vi "Condition Based on Measurement Result.vi"() -> ()   [LabVIEW 2019]
uses:
  <vilib>/DAQmx/read.llb/DAQmx Read (Analog Wfm 1Chan NSamp).vi
  <vilib>/DAQmx/create/channels.llb/DAQmx Create Channel (AI-Temperature-Thermocouple).vi
  <vilib>/DAQmx/configure/timing.llb/DAQmx Timing (Sample Clock).vi
  <vilib>/DAQmx/miscellaneous.llb/DAQmx Fill In Error Info.vi
  <resource>/objmgr/daqmx.rc
panel:
  in  "Stop":bool
  out "Actual Sample Rate (Hz)":dbl
  in  "DAQmx Physical Channel":tag="PCI-6221/ai1"
  out "Last exceeded temperature":waveform(dbl)(graph)={"t0"=timestamp(3640236029.6826963 s since 1904-01-01), "dt"=0.00039059999999999995, "Y"=array[256 elements], "attributes"=variant("NI_ChannelName"=variant(string "PCI-6221/ai0"), "NI_UnitDescription"=variant(string "Deg C"))}
  out "Current temperature":waveform(dbl)(graph)={"t0"=timestamp(3640236029.6826963 s since 1904-01-01), "dt"=0.00039059999999999995, "Y"=array[256 elements], "attributes"=variant("NI_ChannelName"=variant(string "PCI-6221/ai0"), "NI_UnitDescription"=variant(string "Deg C"))}
  in  "Temperature threshold (C)":dbl=30.0
  in  "Number of Samples":i32=256
  in  "Desired Sample Rate (Hz)":dbl=2560.0
  # "Channel Settings"
  # "______________________________________________"
  # "Timing Settings"
  # "______________________________________________"
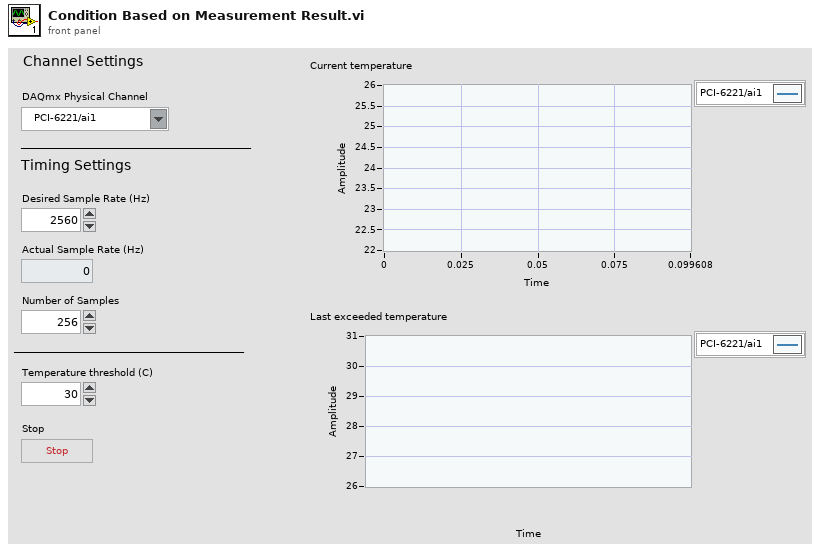
[diagram p1: front panel]
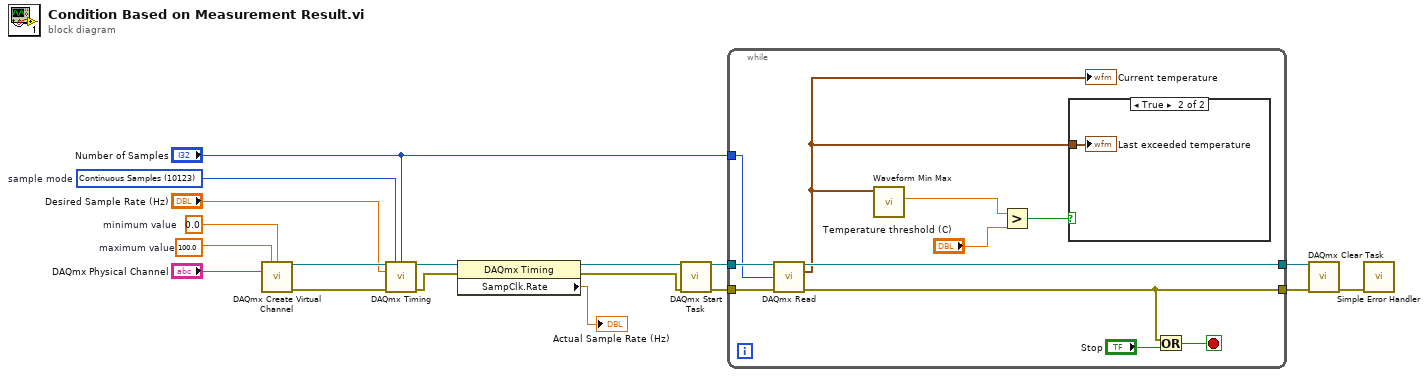
[diagram p0: block diagram]
diagram:
  w8 = 100.0  # maximum value
  w9 = 0.0  # minimum value
  w10 = 10123 items=["Finite Samples"=10178, "Continuous Samples"=10123, "Hardware Timed Single Point"=12522]  # sample mode
  n1 = call-poly <vilib>:"DAQmx Create Virtual Channel.vi"("maximum value"=w8, "minimum value"=w9, "physical channels"="DAQmx Physical Channel") -> ("task out"=w18:refnum<k21>, "error out"=w17:errorcluster)  [unwired: 11 in]
  n2 = call-poly <vilib>:"DAQmx Timing.vi"("task/channels in"=w18, "sample mode"=w10, "samples per channel"="Number of Samples", "rate"="Desired Sample Rate (Hz)", "error in"=w17) -> ("task out"=w15:refnum<k21>, "error out"=w16:errorcluster)  [unwired: 9 in]
  n3 = property class="DAQmx Timing"(reference=w15, error in=w16) -> (reference out=w14:refnum<k21>, error out=w13:errorcluster, "SampClk.Rate"=→"Actual Sample Rate (Hz)":dbl)
  n4 = call <vilib>:"DAQmx Start Task.vi"("task/channels in"=w14, "error in"=w13) -> ("task out"=w12:refnum<k21>, "error out"=w11:errorcluster)  [unwired: 12 in]
  n5 = while {
    tunnel: w12 -> [w29]
    tunnel: w11 -> [w28]
    tunnel: "Number of Samples" -> [w20]
    tunnel: [w27] -> w7
    tunnel: [w26] -> w6
    stop <- w25 stop-if-true
    n6 = call-poly <vilib>:"DAQmx Read.vi"("task/channels in"=w29, "number of samples per channel"=w20, "error in"=w28) -> ("task out"=w27:refnum<k21>, "data"=w21:waveform(dbl), "error out"=w26:errorcluster)  [unwired: 10 in]
    "Current temperature" <- w21
    n7 = call <vilib>:"Waveform Min Max.vi"("waveform in"=w21) -> ("Y max"=w24:dbl)  [unwired: 5 in, 5 out]
    n8 = Greater?(x=w24, y="Temperature threshold (C)") -> (0:w23:bool)
    n9 = case shown="True" w23 {
      tunnel: w21 -> [_ w30]
      frame False {
      }
      frame True {
        "Last exceeded temperature" <- w30
      }
    }
    n10 = Or(x=w26, y="Stop") -> (x .or. y?=w25:bool)
  }
  n11 = call <vilib>:"DAQmx Clear Task.vi"("task in"=w7, "error in"=w6) -> ("error out"=w5:errorcluster)  [unwired: 13 in]
  n12 = call <vilib>:"Simple Error Handler.vi"("error in (no error)"=w5) -> ()  [unwired: 4 in, 5 out]
